vi "Queue References FGV.vi"(8 "error in":errorcluster, 11 "function":enum16{"obtain", "get", "release"}(ring)) -> (0 "error out":errorcluster, 3 "module queues":T1)   [LabVIEW 2017, in "Logger.lvlib"]
uses:
  Logger.lvlib
  Private TypeDefs/Module Queues.ctl
  Private TypeDefs/Message Queue Element.ctl
  Global TypeDefs/Registered Modules.ctl
  Private TypeDefs/Messages.ctl
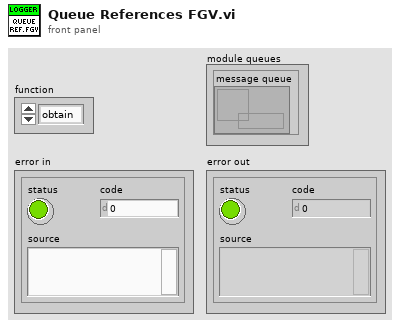
[diagram p1: front panel]
types:
  T1 = typedef "Logger.lvlib/Module Queues.ctl" = cluster{"message queue":refnum<queue>}
  T2 = typedef "Logger.lvlib/Message Queue Element.ctl" = cluster{"source":T3, "message":T4, "data":variant}
  T3 = typedef "Registered Modules.ctl" = enum16{"Controller", "DAQ", "Error Handler", "Game", "myPAM", "WinHost", "Logger"}
  T4 = typedef "Logger.lvlib/Messages.ctl" = enum16{"log event", "shutdown"}
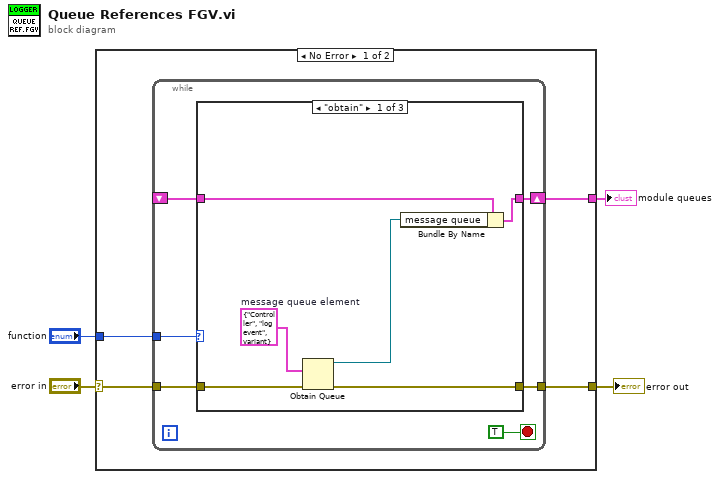
[diagram p0: block diagram]
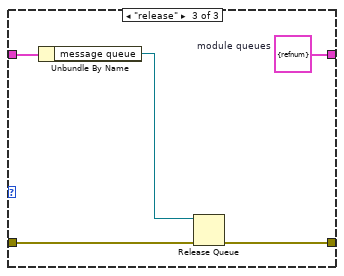
[diagram p3: hidden frame]
diagram:
  n1 = case shown="No Error" "error in" {
    selector: "error in" -> [w8 w28]
    tunnel: [w7 w28] -> w3
    tunnel: "function" -> [w6 _]
    tunnel: [w5 _] -> w1
    frame No Error {
      n2 = while {
        tunnel: w8 -> [w13]
        tunnel: [w12] -> w7
        tunnel: w6 -> [w11]
        shift-right: [w10] -> w5
        shift-left: _ -> [w9]
        stop <- TRUE stop-if-true
        n3 = case shown="\"obtain\"" w11 {
          tunnel: w13 -> [w20 w22 w27]
          tunnel: [w18 w22 w26] -> w12
          tunnel: [w15 w21 w23] -> w10
          tunnel: w9 -> [w17 w21 w25]
          frame "obtain" {
            w19 = T2 {"source"=enum."Controller", "message"=enum."log event", "data"=variant}  # message queue element
            n4 = Obtain Queue(element data type=w19, error in (no error)=w20) -> (queue out=w16:refnum<queue>, error out=w18:errorcluster)  [unwired: 3 in, 1 out]
            n5 = Bundle By Name(cluster=w17, "message queue"=w16) -> (w15:T1)
          }
          frame "get", Default {
          }
          frame "release" {
            w23 = T1 {"message queue"=refnum}  # module queues
            n6 = Unbundle By Name(w25) -> ("message queue"=w24:refnum<queue>)
            n7 = Release Queue(queue=w24, error in (no error)=w27) -> (error out=w26:errorcluster)  [unwired: 1 in, 2 out]
          }
        }
      }
    }
    frame Error {
    }
  }
  "error out" <- w3
  "module queues" <- w1
